vi "ClusterDemo-BinaryConversion.vi"() -> ()   [LabVIEW 2018]
panel:
  out "Input Cluster 2":cluster{"8":bool, "4":bool, "2":bool, "1":bool}
  in  "Input Cluster":cluster{"8":bool, "4":bool, "2":bool, "1":bool}
  # "Binary to Decimal Number Converter"
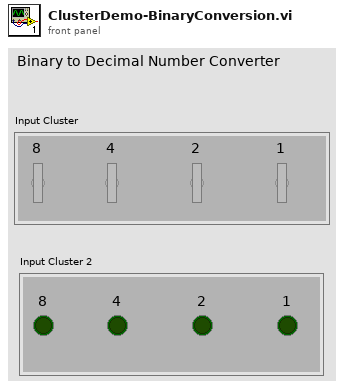
[diagram p1: front panel]
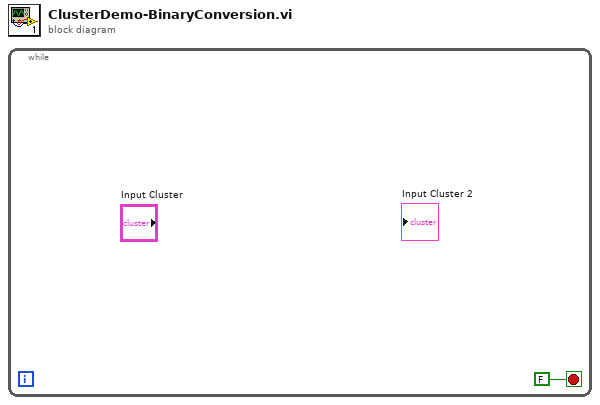
[diagram p0: block diagram]
diagram:
  n1 = while {
    stop <- FALSE stop-if-true
  }
